vi "战舰弹窗.vi"() -> ()   [LabVIEW 2018]
panel:
  in  "关卡":dbl
  out "失败界面":picture
  out "胜利界面":picture
  out "敌机是否入侵":bool
  out "得分":dbl
  out "战舰爆炸":picture
  out "血量":dbl
  out "战舰血量":T1 scale=0.0..100.0
  out "敌机爆炸":picture
  in  "敌机数量":dbl
  in  "敌机速度":dbl
  out "敌机":picture
  out "按键":dbl
  out "战舰":T2
  out "激光武器1":T3
  out "激光武器 2":T3
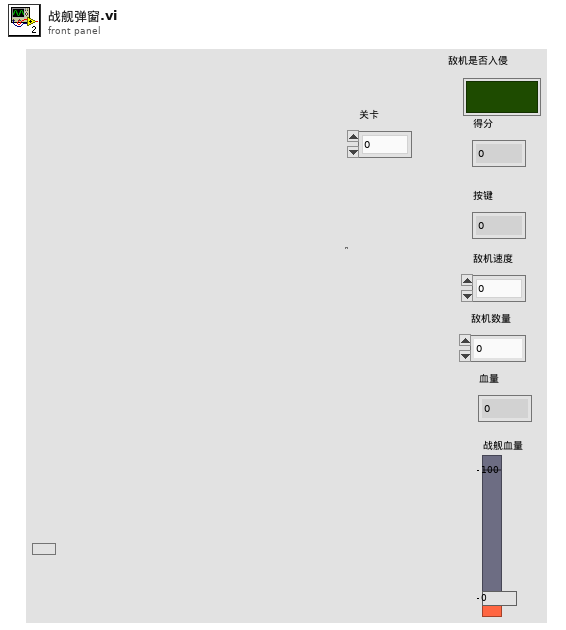
[diagram p1: front panel]
types:
  T1 = typedef "战列巡洋舰_血条.ctl" = dbl
  T2 = typedef "战列巡洋舰.ctl" = picture
  T3 = typedef "战列巡洋舰_激光武器.ctl" = picture
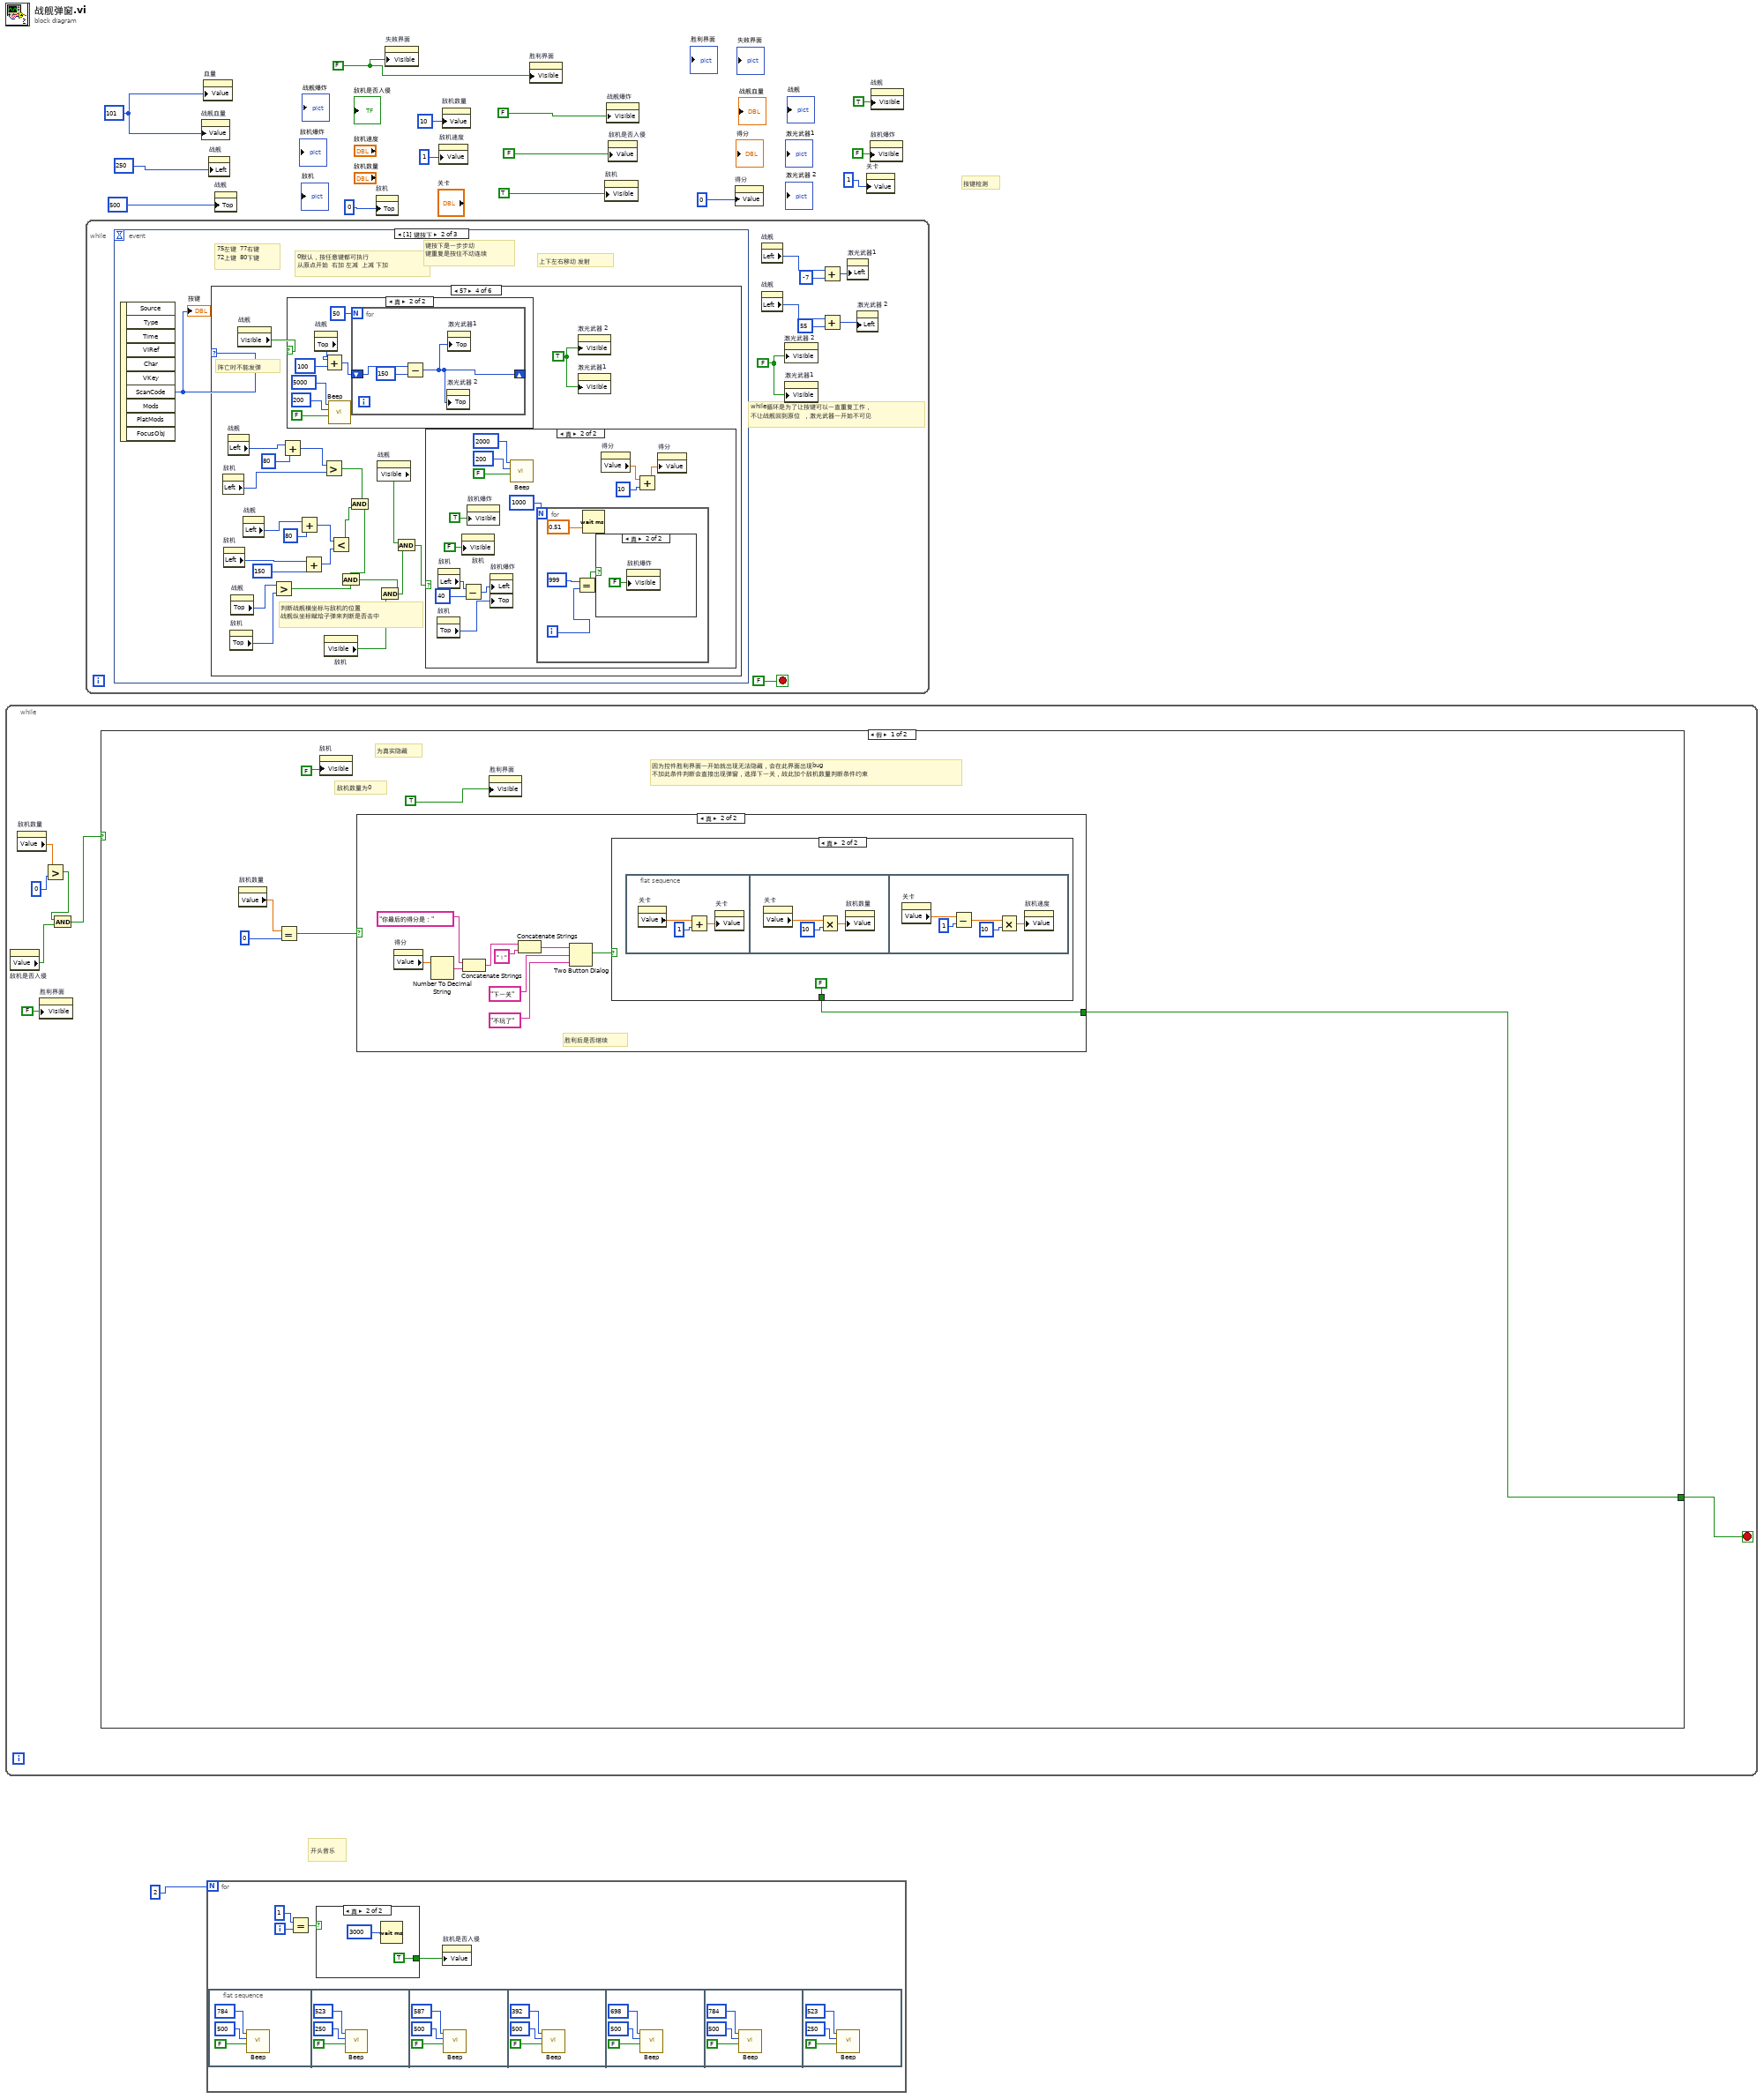
[diagram p0: block diagram]
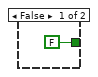
[diagram p2: hidden frame]
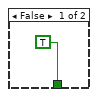
[diagram p4: hidden frame]
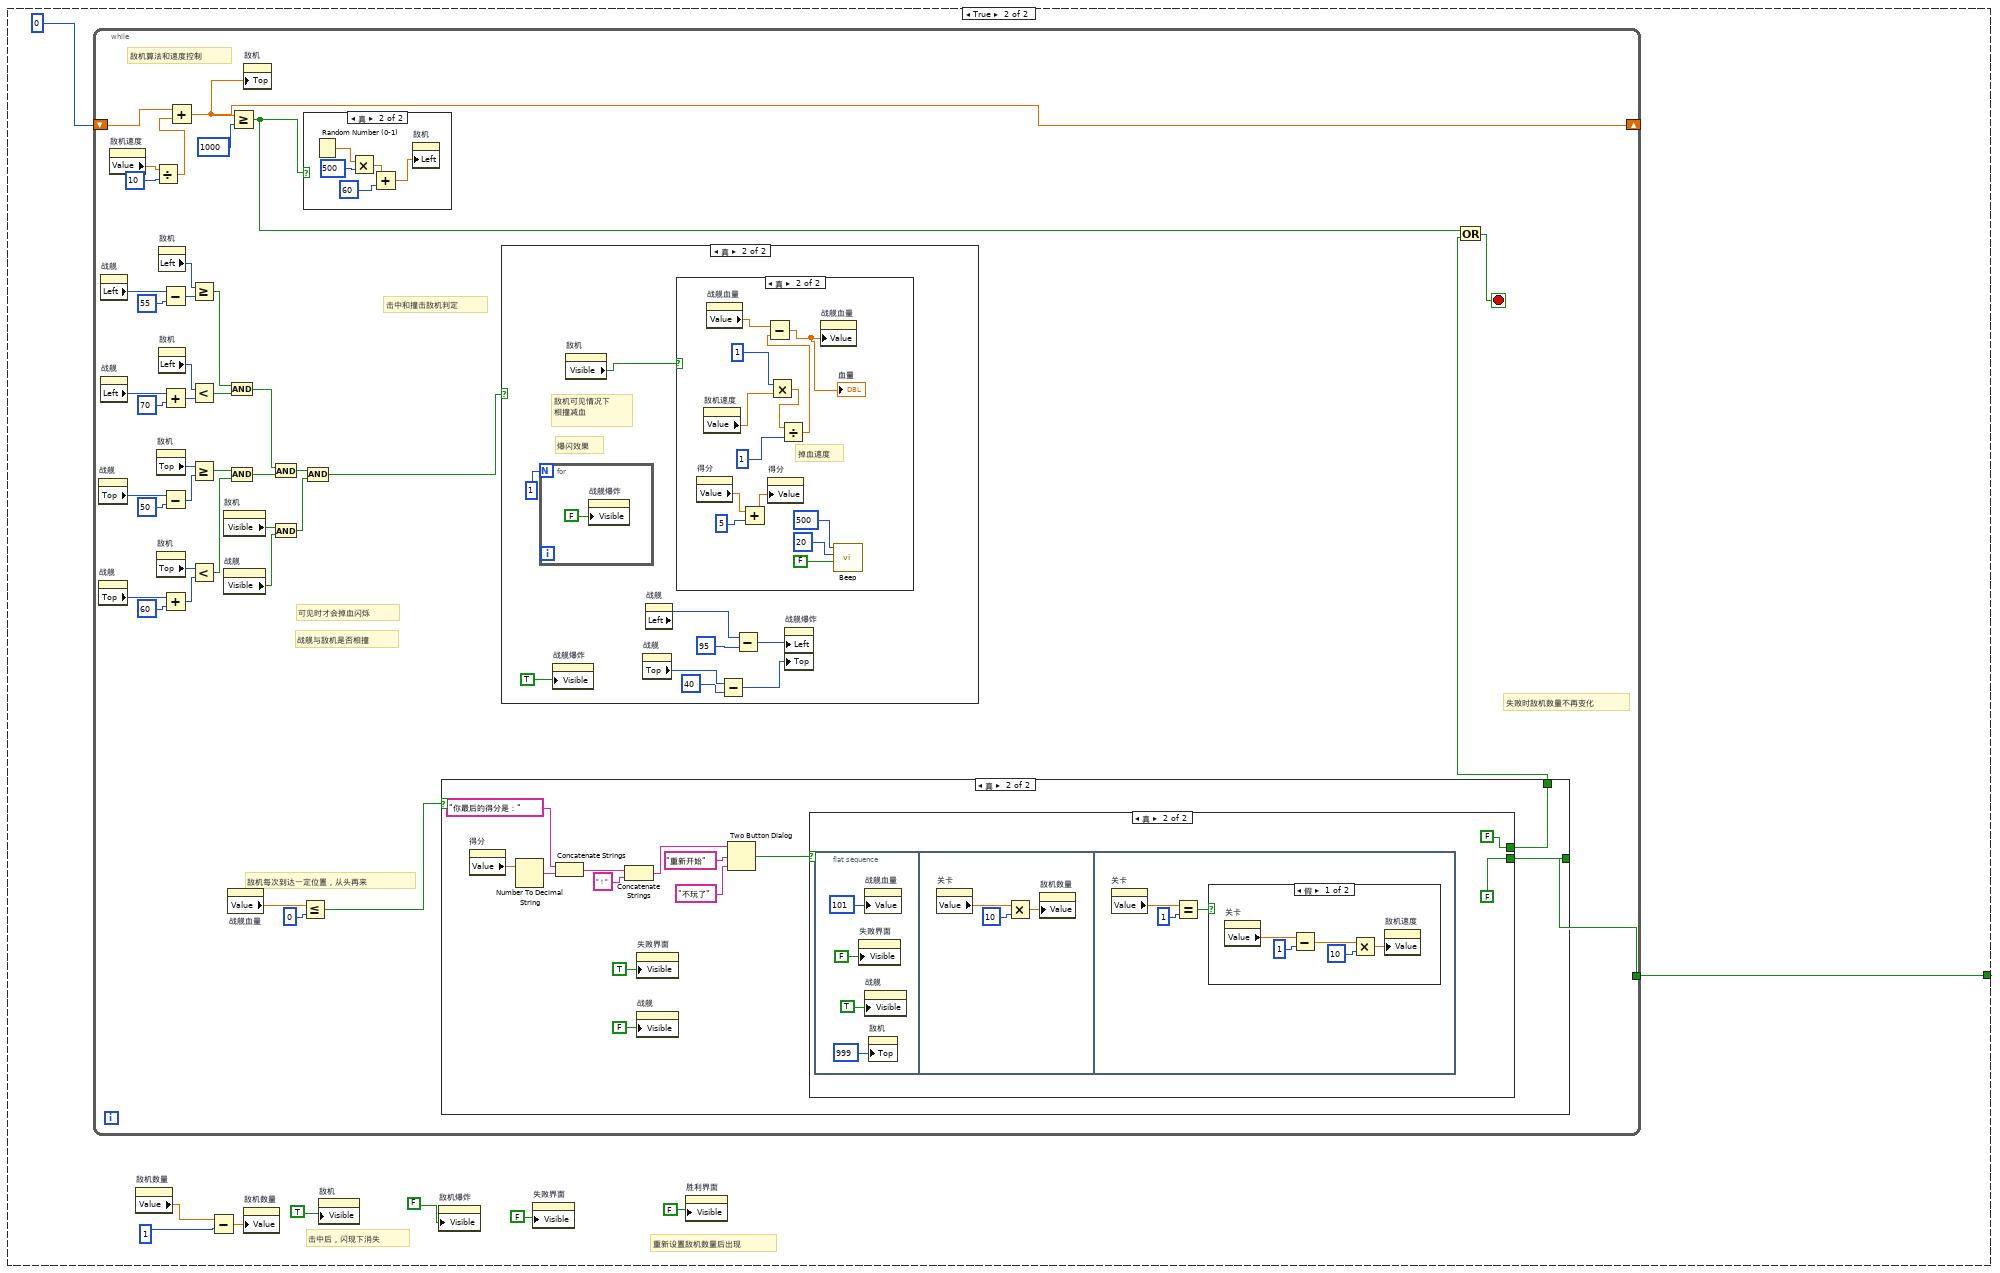
[diagram p5: hidden frame]
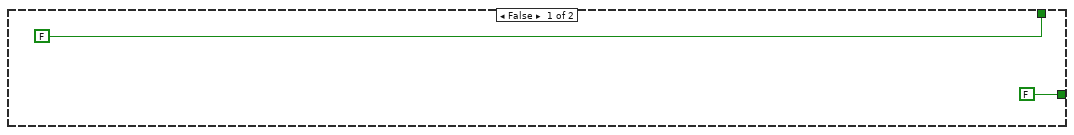
[diagram p6: hidden frame]
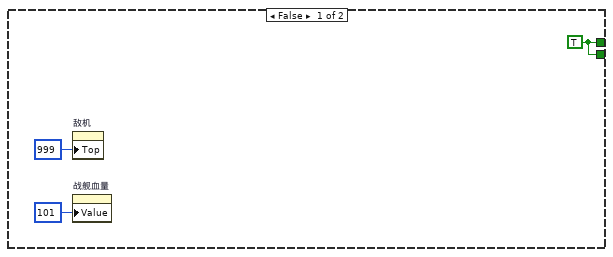
[diagram p7: hidden frame]
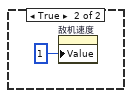
[diagram p8: hidden frame]
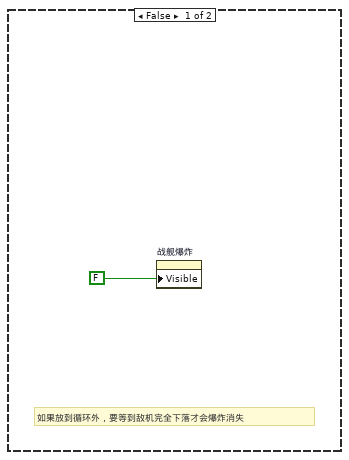
[diagram p9: hidden frame]
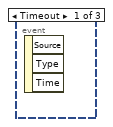
[diagram p12: hidden frame]
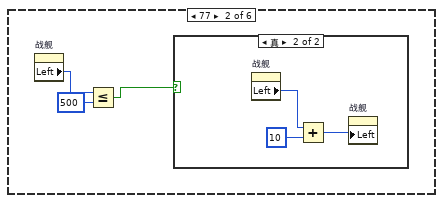
[diagram p14: hidden frame]
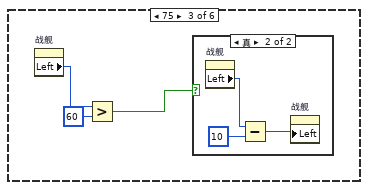
[diagram p16: hidden frame]
diagram:
  w1 = FALSE ("可见")
  w9 = 101
  # "开头音乐"
  # "按键检测"
  n1 = while {
    stop <- w17 stop-if-true
    n2 = property on="敌机是否入侵" class="Bool (严格)"() -> ("Value"=w20:bool)  [unwired: 2 in, 2 out]
    n3 = property on="敌机数量" class="DigNum (严格)"() -> ("Value"=w22:dbl)  [unwired: 2 in, 2 out]
    n4 = property on="胜利界面" class="Pict"("Visible"=FALSE ("可见")) -> ()  [unwired: 2 in, 2 out]
    n5 = Greater?(x=w22, y=0) -> (0:w19:bool)
    n6 = And(x=w19, y=w20) -> (x .and. y?=w18:bool)
    n7 = case shown="假" w18 {
      tunnel: [w26 w53] -> w17
      frame False {
        # "因为控件胜利界面一开始就出现无法隐藏，会在此界面出现bug\n不加此条件判断会直接出现弹窗，选择下一关，故此加个敌机数量判断条件约束"
        # "敌机数量为0"
        # "为真实隐藏"
        n8 = property on="敌机数量" class="DigNum (严格)"() -> ("Value"=w25:dbl)  [unwired: 2 in, 2 out]
        n9 = Equal?(x=w25, y=0) -> (x = y?=w23:bool)
        n10 = property on="敌机" class="Pict"("Visible"=FALSE ("可见")) -> ()  [unwired: 2 in, 2 out]
        n11 = case shown="真" w23 {
          tunnel: [_ w29] -> w26
          frame False {
          }
          frame True {
            # "胜利后是否继续"
            n12 = property on="得分" class="DigNum (严格)"() -> ("Value"=w37:dbl)  [unwired: 2 in, 2 out]
            n13 = Number To Decimal String(number=w37) -> (decimal integer string=w35:string)  [unwired: 1 in]
            n14 = Concatenate Strings("你最后的得分是：", w35) -> (w34:string)
            n15 = Concatenate Strings(w34, "！") -> (w32:string)
            n16 = Two Button Dialog(message=w32, 1:"不玩了" ("F按钮名称（“取消”）"), 2:"下一关" ("T按钮名称（“确定”）")) -> (T button?=w38:bool)
            n17 = case shown="真" w38 {
              tunnel: [TRUE FALSE] -> w29
              frame False {
              }
              frame True {
                n18 = flat-sequence {
                  frame #0 {
                    n19 = property on="关卡" class="DigNum (严格)"() -> ("Value"=w43:dbl)  [unwired: 2 in, 2 out]
                    n20 = Add(x=w43, y=1) -> (x+y=w41:dbl)
                    n21 = property on="关卡" class="DigNum (严格)"("Value"=w41) -> ()  [unwired: 2 in, 2 out]
                  }
                  frame #1 {
                    n22 = property on="关卡" class="DigNum (严格)"() -> ("Value"=w45:dbl)  [unwired: 2 in, 2 out]
                    n23 = Multiply(x=w45, y=10) -> (x*y=w46:dbl)
                    n24 = property on="敌机数量" class="DigNum (严格)"("Value"=w46) -> ()  [unwired: 2 in, 2 out]
                  }
                  frame #2 {
                    n25 = property on="关卡" class="DigNum (严格)"() -> ("Value"=w50:dbl)  [unwired: 2 in, 2 out]
                    n26 = Subtract(x=w50, y=1) -> (x-y=w48:dbl)
                    n27 = Multiply(x=w48, y=10) -> (x*y=w47:dbl)
                    n28 = property on="敌机速度" class="DigNum (严格)"("Value"=w47) -> ()  [unwired: 2 in, 2 out]
                  }
                }
              }
            }
          }
        }
        n29 = property on="胜利界面" class="Pict"("Visible"=TRUE ("可见")) -> ()  [unwired: 2 in, 2 out]
      }
      frame True {
        # "重新设置敌机数量后出现"
        # "击中后，闪现下消失"
        # "敌机每次到达一定位置，从头再来"
        n30 = while {
          shift-right: [w98] -> _
          shift-left: 0 -> [w100]
          tunnel: [w64] -> w53
          stop <- w62 stop-if-true
          # "失败时敌机数量不再变化"
          # "击中和撞击敌机判定"
          # "可见时才会掉血闪烁"
          # "战舰与敌机是否相撞"
          # "敌机算法和速度控制"
          n31 = property on="战舰" class="Pict (严格)"() -> ("Top"=w83:i32)  [unwired: 2 in, 2 out]
          n32 = property on="战舰" class="Pict (严格)"() -> ("Top"=w77:i32)  [unwired: 2 in, 2 out]
          n33 = property on="战舰" class="Pict (严格)"() -> ("Left"=w93:i32)  [unwired: 2 in, 2 out]
          n34 = property on="战舰" class="Pict (严格)"() -> ("Left"=w87:i32)  [unwired: 2 in, 2 out]
          n35 = property on="敌机速度" class="DigNum (严格)"() -> ("Value"=w97:dbl)  [unwired: 2 in, 2 out]
          n36 = Divide(x=w97, y=10) -> (x/y=w96:dbl)
          n37 = property on="敌机" class="Pict"() -> ("Top"=w84:i32)  [unwired: 2 in, 2 out]
          n38 = property on="敌机" class="Pict"() -> ("Top"=w76:i32)  [unwired: 2 in, 2 out]
          n39 = property on="敌机" class="Pict"() -> ("Left"=w94:i32)  [unwired: 2 in, 2 out]
          n40 = property on="敌机" class="Pict"() -> ("Left"=w89:i32)  [unwired: 2 in, 2 out]
          n41 = Subtract(x=w93, y=55) -> (x-y=w92:i32)
          n42 = Add(x=w87, y=70) -> (x+y=w86:i32)
          n43 = Subtract(x=w83, y=50) -> (x-y=w81:i32)
          n44 = Add(x=w77, y=60) -> (x+y=w79:i32)
          n45 = Add(x=w100, y=w96) -> (x+y=w98:dbl)
          n46 = Greater Or Equal?(x=w94, y=w92) -> (x >= y?=w90:bool)
          n47 = Less?(x=w89, y=w86) -> (x < y?=w85:bool)
          n48 = Greater Or Equal?(x=w84, y=w81) -> (x >= y?=w75:bool)
          n49 = Less?(x=w76, y=w79) -> (x < y?=w74:bool)
          n50 = property on="敌机" class="Pict"() -> ("Visible"=w67:bool)  [unwired: 2 in, 2 out]
          n51 = property on="战舰" class="Pict (严格)"() -> ("Visible"=w66:bool)  [unwired: 2 in, 2 out]
          n52 = And(x=w90, y=w85) -> (x .and. y?=w80:bool)
          n53 = And(x=w75, y=w74) -> (x .and. y?=w73:bool)
          n54 = property on="战舰血量" class="Slide (严格)"() -> ("Value"=w69:T1)  [unwired: 2 in, 2 out]
          n55 = Greater Or Equal?(x=w98, y=1000) -> (x >= y?=w63:bool)
          n56 = property on="敌机" class="Pict"("Top"=w98) -> ()  [unwired: 2 in, 2 out]
          n57 = And(x=w80, y=w73) -> (x .and. y?=w72:bool)
          n58 = And(x=w67, y=w66) -> (x .and. y?=w65:bool)
          n59 = Less Or Equal?(x=w69, y=0) -> (x <= y?=w70:bool)
          n60 = case shown="真" w63 {
            frame False {
            }
            frame True {
              n61 = Random Number (0-1)() -> (number: 0 to 1=w165:dbl)
              n62 = Multiply(x=w165, y=500) -> (x*y=w163:dbl)
              n63 = Add(x=w163, y=60) -> (x+y=w162:dbl)
              n64 = property on="敌机" class="Pict"("Left"=w162) -> ()  [unwired: 2 in, 2 out]
            }
          }
          n65 = And(x=w72, y=w65) -> (x .and. y?=w71:bool)
          n66 = case shown="真" w70 {
            tunnel: [FALSE w104] -> w64
            tunnel: [FALSE w103] -> w61
            frame False {
            }
            frame True {
              n67 = property on="得分" class="DigNum (严格)"() -> ("Value"=w115:dbl)  [unwired: 2 in, 2 out]
              n68 = Number To Decimal String(number=w115) -> (decimal integer string=w114:string)  [unwired: 1 in]
              n69 = Concatenate Strings("你最后的得分是：", w114) -> (w113:string)
              n70 = Concatenate Strings(w113, "！") -> (w112:string)
              n71 = property on="失败界面" class="Pict"("Visible"=TRUE ("可见")) -> ()  [unwired: 2 in, 2 out]
              n72 = property on="战舰" class="Pict (严格)"("Visible"=FALSE ("可见")) -> ()  [unwired: 2 in, 2 out]
              n73 = Two Button Dialog(message=w112, 1:"不玩了" ("F按钮名称（“取消”）"), 2:"重新开始" ("T按钮名称（“确定”）")) -> (T button?=w107:bool)
              n74 = case shown="真" w107 {
                tunnel: [w116 FALSE] -> w104
                tunnel: [w116 FALSE] -> w103
                frame False {
                  w116 = TRUE
                  n75 = property on="敌机" class="Pict"("Top"=999 ("位置:置顶")) -> ()  [unwired: 2 in, 2 out]
                  n76 = property on="战舰血量" class="Slide (严格)"("Value"=101) -> ()  [unwired: 2 in, 2 out]
                }
                frame True {
                  n77 = flat-sequence {
                    frame #0 {
                      n78 = property on="失败界面" class="Pict"("Visible"=FALSE ("可见")) -> ()  [unwired: 2 in, 2 out]
                      n79 = property on="战舰血量" class="Slide (严格)"("Value"=101) -> ()  [unwired: 2 in, 2 out]
                      n80 = property on="战舰" class="Pict (严格)"("Visible"=TRUE ("可见")) -> ()  [unwired: 2 in, 2 out]
                      n81 = property on="敌机" class="Pict"("Top"=999 ("位置:置顶")) -> ()  [unwired: 2 in, 2 out]
                    }
                    frame #1 {
                      n82 = property on="关卡" class="DigNum (严格)"() -> ("Value"=w125:dbl)  [unwired: 2 in, 2 out]
                      n83 = Multiply(x=w125, y=10) -> (x*y=w127:dbl)
                      n84 = property on="敌机数量" class="DigNum (严格)"("Value"=w127) -> ()  [unwired: 2 in, 2 out]
                    }
                    frame #2 {
                      n85 = property on="关卡" class="DigNum (严格)"() -> ("Value"=w130:dbl)  [unwired: 2 in, 2 out]
                      n86 = Equal?(x=w130, y=1) -> (x = y?=w128:bool)
                      n87 = case shown="假" w128 {
                        frame False {
                          n88 = property on="关卡" class="DigNum (严格)"() -> ("Value"=w134:dbl)  [unwired: 2 in, 2 out]
                          n89 = Subtract(x=w134, y=1) -> (x-y=w131:dbl)
                          n90 = Multiply(x=w131, y=10) -> (x*y=w135:dbl)
                          n91 = property on="敌机速度" class="DigNum (严格)"("Value"=w135) -> ()  [unwired: 2 in, 2 out]
                        }
                        frame True {
                          n92 = property on="敌机速度" class="DigNum (严格)"("Value"=1) -> ()  [unwired: 2 in, 2 out]
                        }
                      }
                    }
                  }
                }
              }
            }
          }
          n93 = case shown="真" w71 {
            frame False {
              # "如果放到循环外，要等到敌机完全下落才会爆炸消失"
              n94 = property on="战舰爆炸" class="Pict"("Visible"=FALSE ("可见")) -> ()  [unwired: 2 in, 2 out]
            }
            frame True {
              # "爆闪效果"
              # "敌机可见情况下\n相撞减血"
              n95 = for {
                N: 1 -> [_]
                n96 = property on="战舰爆炸" class="Pict"("Visible"=FALSE ("可见")) -> ()  [unwired: 2 in, 2 out]
              }
              n97 = property on="战舰爆炸" class="Pict"("Visible"=TRUE ("可见")) -> ()  [unwired: 2 in, 2 out]
              n98 = property on="敌机" class="Pict"() -> ("Visible"=w146:bool)  [unwired: 2 in, 2 out]
              n99 = property on="战舰" class="Pict (严格)"() -> ("Top"=w141:i32)  [unwired: 2 in, 2 out]
              n100 = property on="战舰" class="Pict (严格)"() -> ("Left"=w144:i32)  [unwired: 2 in, 2 out]
              n101 = case shown="真" w146 {
                frame False {
                }
                frame True {
                  # "掉血速度"
                  n102 = property on="得分" class="DigNum (严格)"() -> ("Value"=w153:dbl)  [unwired: 2 in, 2 out]
                  n103 = property on="敌机速度" class="DigNum (严格)"() -> ("Value"=w159:dbl)  [unwired: 2 in, 2 out]
                  n104 = property on="战舰血量" class="Slide (严格)"() -> ("Value"=w160:T1)  [unwired: 2 in, 2 out]
                  n105 = Add(x=w153, y=5) -> (x+y=w152:dbl)
                  n106 = Multiply(x=1, y=w159) -> (x*y=w158:dbl)
                  n107 = property on="得分" class="DigNum (严格)"("Value"=w152) -> ()  [unwired: 2 in, 2 out]
                  n108 = Divide(x=w158, y=1) -> (x/y=w155:dbl)
                  n109 = Subtract(x=w160, y=w155) -> (x-y=w154:T1)
                  "血量" <- w154
                  n110 = property on="战舰血量" class="Slide (严格)"("Value"=w154) -> ()  [unwired: 2 in, 2 out]
                  n111 = call <vilib>:"Beep.vi"("use system alert? (T)"=FALSE, "duration (msec)"=u32 20, "frequency (Hz)"=u32 500) -> ()  [unwired: 9 in]
                }
              }
              n112 = Subtract(x=w141, y=40) -> (x-y=w139:i32)
              n113 = Subtract(x=w144, y=95) -> (x-y=w142:i32)
              n114 = property on="战舰爆炸" class="Pict"("Left"=w142, "Top"=w139) -> ()  [unwired: 2 in, 2 out]
            }
          }
          n115 = Or(x=w63, y=w61) -> (x .or. y?=w62:bool)
        }
        n116 = property on="敌机数量" class="DigNum (严格)"() -> ("Value"=w58:dbl)  [unwired: 2 in, 2 out]
        n117 = Subtract(x=w58, y=1) -> (x-y=w59:dbl)
        n118 = property on="敌机数量" class="DigNum (严格)"("Value"=w59) -> ()  [unwired: 2 in, 2 out]
        n119 = property on="敌机" class="Pict"("Visible"=TRUE ("可见")) -> ()  [unwired: 2 in, 2 out]
        n120 = property on="敌机爆炸" class="Pict"("Visible"=FALSE ("可见")) -> ()  [unwired: 2 in, 2 out]
        n121 = property on="失败界面" class="Pict"("Visible"=FALSE ("可见")) -> ()  [unwired: 2 in, 2 out]
        n122 = property on="胜利界面" class="Pict"("Visible"=FALSE ("可见")) -> ()  [unwired: 2 in, 2 out]
      }
    }
  }
  n123 = while {
    stop <- FALSE stop-if-true
    w166 = FALSE
    # "while循环是为了让按键可以一直重复工作，\n不让战舰回到原位  ，激光武器一开始不可见"
    n124 = event shown="[1] 键按下" {
      selector: _ -> [_ _ _]
      dyn-events: _ -> [_ _ _]
      timeout: _ -> [_ _ _]
      event Timeout {
        n125 = event-data() -> ()  [unwired: 1 in, 3 out]
      }
      event Key Down {
        # "上下左右移动 发射"
        # "键按下是一步步动\n键重复是按住不动连续"
        # "75左键  77右键\n72上键  80下键"
        # "0默认，按任意键都可执行\n从原点开始  右加 左减  上减 下加"
        n126 = event-data() -> ("ScanCode"=w174:i16)  [unwired: 1 in, 9 out]
        "按键" <- w174
        n127 = case shown="57" w174 {
          frame 0, Default {
          }
          frame 77 {
            n128 = property on="战舰" class="Pict (严格)"() -> ("Left"=w177:i32)  [unwired: 2 in, 2 out]
            n129 = Less Or Equal?(x=w177, y=500) -> (x <= y?=w175:bool)
            n130 = case shown="真" w175 {
              frame False {
              }
              frame True {
                n131 = property on="战舰" class="Pict (严格)"() -> ("Left"=w179:i32)  [unwired: 2 in, 2 out]
                n132 = Add(x=w179, y=10) -> (x+y=w180:i32)
                n133 = property on="战舰" class="Pict (严格)"("Left"=w180) -> ()  [unwired: 2 in, 2 out]
              }
            }
          }
          frame 75 {
            n134 = property on="战舰" class="Pict (严格)"() -> ("Left"=w183:i32)  [unwired: 2 in, 2 out]
            n135 = Greater?(x=w183, y=60) -> (0:w181:bool)
            n136 = case shown="真" w181 {
              frame False {
              }
              frame True {
                n137 = property on="战舰" class="Pict (严格)"() -> ("Left"=w185:i32)  [unwired: 2 in, 2 out]
                n138 = Subtract(x=w185, y=10) -> (x-y=w186:i32)
                n139 = property on="战舰" class="Pict (严格)"("Left"=w186) -> ()  [unwired: 2 in, 2 out]
              }
            }
          }
          frame 57 {
            w209 = TRUE
            # "阵亡时不能发弹"
            # "判断战舰横坐标与敌机的位置\n战舰纵坐标赋给子弹来判断是否击中"
            n140 = property on="敌机" class="Pict"() -> ("Left"=w206:i32)  [unwired: 2 in, 2 out]
            n141 = property on="敌机" class="Pict"() -> ("Left"=w199:i32)  [unwired: 2 in, 2 out]
            n142 = property on="战舰" class="Pict (严格)"() -> ("Left"=w208:i32)  [unwired: 2 in, 2 out]
            n143 = property on="敌机" class="Pict"() -> ("Top"=w193:i32)  [unwired: 2 in, 2 out]
            n144 = property on="战舰" class="Pict (严格)"() -> ("Top"=w194:i32)  [unwired: 2 in, 2 out]
            n145 = property on="战舰" class="Pict (严格)"() -> ("Visible"=w187:bool)  [unwired: 2 in, 2 out]
            n146 = property on="战舰" class="Pict (严格)"() -> ("Left"=w201:i32)  [unwired: 2 in, 2 out]
            n147 = Greater?(x=w194, y=w193) -> (0:w195:bool)
            n148 = Add(x=w208, y=80) -> (x+y=w205:i32)
            n149 = case shown="真" w187 {
              frame False {
              }
              frame True {
                n150 = property on="战舰" class="Pict (严格)"() -> ("Top"=w215:i32)  [unwired: 2 in, 2 out]
                n151 = Add(x=w215, y=100) -> (x+y=w213:i32)
                n152 = call <vilib>:"Beep.vi"("use system alert? (T)"=FALSE, "duration (msec)"=u32 200, "frequency (Hz)"=u32 5000) -> ()  [unwired: 9 in]
                n153 = for {
                  N: 50 -> [_]
                  shift-right: [w217] -> _
                  shift-left: w213 -> [w219]
                  n154 = Subtract(x=w219, y=150) -> (x-y=w217:i32)
                  n155 = property on="激光武器 2" class="Pict (严格)"("Top"=w217) -> ()  [unwired: 2 in, 2 out]
                  n156 = property on="激光武器1" class="Pict (严格)"("Top"=w217) -> ()  [unwired: 2 in, 2 out]
                }
              }
            }
            n157 = Add(x=w201, y=80) -> (x+y=w203:i32)
            n158 = Add(x=w199, y=150) -> (x+y=w198:i32)
            n159 = Greater?(x=w205, y=w206) -> (0:w204:bool)
            n160 = property on="敌机" class="Pict"() -> ("Visible"=w191:bool)  [unwired: 2 in, 2 out]
            n161 = Less?(x=w203, y=w198) -> (x < y?=w200:bool)
            n162 = And(x=w204, y=w200) -> (x .and. y?=w196:bool)
            n163 = And(x=w196, y=w195) -> (x .and. y?=w192:bool)
            n164 = property on="战舰" class="Pict (严格)"() -> ("Visible"=w190:bool)  [unwired: 2 in, 2 out]
            n165 = And(x=w192, y=w191) -> (x .and. y?=w189:bool)
            n166 = And(x=w190, y=w189) -> (x .and. y?=w188:bool)
            n167 = case shown="真" w188 {
              frame False {
              }
              frame True {
                n168 = property on="敌机" class="Pict"() -> ("Top"=w230:i32)  [unwired: 2 in, 2 out]
                n169 = property on="敌机" class="Pict"() -> ("Left"=w228:i32)  [unwired: 2 in, 2 out]
                n170 = property on="敌机" class="Pict"("Visible"=FALSE ("可见")) -> ()  [unwired: 2 in, 2 out]
                n171 = Subtract(x=w228, y=40) -> (x-y=w227:i32)
                n172 = property on="敌机爆炸" class="Pict"("Visible"=TRUE ("可见")) -> ()  [unwired: 2 in, 2 out]
                n173 = property on="敌机爆炸" class="Pict"("Left"=w227, "Top"=w230) -> ()  [unwired: 2 in, 2 out]
                n174 = call <vilib>:"Beep.vi"("use system alert? (T)"=FALSE, "duration (msec)"=u32 200, "frequency (Hz)"=u32 2000) -> ()  [unwired: 9 in]
                n175 = for {
                  N: 1000 -> [_]
                  i -> [w235]
                  n176 = Equal?(x=999, y=w235) -> (x = y?=w236:bool)
                  n177 = Wait (ms)(milliseconds to wait=0.51) -> ()  [unwired: 1 out]
                  n178 = case shown="真" w236 {
                    frame False {
                    }
                    frame True {
                      n179 = property on="敌机爆炸" class="Pict"("Visible"=FALSE ("可见")) -> ()  [unwired: 2 in, 2 out]
                    }
                  }
                }
                n180 = property on="得分" class="DigNum (严格)"() -> ("Value"=w225:dbl)  [unwired: 2 in, 2 out]
                n181 = Add(x=w225, y=10) -> (x+y=w223:dbl)
                n182 = property on="得分" class="DigNum (严格)"("Value"=w223) -> ()  [unwired: 2 in, 2 out]
              }
            }
            n183 = property on="激光武器 2" class="Pict (严格)"("Visible"=w209) -> ()  [unwired: 2 in, 2 out]
            n184 = property on="激光武器1" class="Pict (严格)"("Visible"=w209) -> ()  [unwired: 2 in, 2 out]
          }
          frame 80 {
            n185 = property on="战舰" class="Pict (严格)"() -> ("Top"=w240:i32)  [unwired: 2 in, 2 out]
            n186 = Less?(x=w240, y=525) -> (x < y?=w238:bool)
            n187 = case shown="真" w238 {
              frame False {
              }
              frame True {
                n188 = property on="战舰" class="Pict (严格)"() -> ("Top"=w242:i32)  [unwired: 2 in, 2 out]
                n189 = Add(x=w242, y=10) -> (x+y=w241:i32)
                n190 = property on="战舰" class="Pict (严格)"("Top"=w241) -> ()  [unwired: 2 in, 2 out]
              }
            }
          }
          frame 72 {
            n191 = property on="战舰" class="Pict (严格)"() -> ("Top"=w246:i32)  [unwired: 2 in, 2 out]
            n192 = Greater Or Equal?(x=w246, y=25) -> (x >= y?=w245:bool)
            n193 = case shown="真" w245 {
              frame False {
              }
              frame True {
                n194 = property on="战舰" class="Pict (严格)"() -> ("Top"=w249:i32)  [unwired: 2 in, 2 out]
                n195 = Subtract(x=w249, y=10) -> (x-y=w248:i32)
                n196 = property on="战舰" class="Pict (严格)"("Top"=w248) -> ()  [unwired: 2 in, 2 out]
              }
            }
          }
        }
      }
      event Key Repeat {
        # "75左键  77右键\n72上键  80下键\n空格 57"
        # "0默认，按任意键都可执行\n从原点开始  右加 左减  上减 下加"
        n197 = event-data() -> ("ScanCode"=w250:i16)  [unwired: 1 in, 9 out]
        n198 = case shown="72" w250 {
          frame 0, Default {
          }
          frame 77 {
            n199 = property on="战舰" class="Pict (严格)"() -> ("Left"=w253:i32)  [unwired: 2 in, 2 out]
            n200 = Less Or Equal?(x=w253, y=500) -> (x <= y?=w252:bool)
            n201 = case shown="真" w252 {
              frame False {
              }
              frame True {
                n202 = property on="战舰" class="Pict (严格)"() -> ("Left"=w255:i32)  [unwired: 2 in, 2 out]
                n203 = Add(x=w255, y=10) -> (x+y=w256:i32)
                n204 = property on="战舰" class="Pict (严格)"("Left"=w256) -> ()  [unwired: 2 in, 2 out]
              }
            }
          }
          frame 75 {
            n205 = property on="战舰" class="Pict (严格)"() -> ("Left"=w259:i32)  [unwired: 2 in, 2 out]
            n206 = Greater Or Equal?(x=w259, y=25) -> (x >= y?=w258:bool)
            n207 = case shown="真" w258 {
              frame False {
              }
              frame True {
                n208 = property on="战舰" class="Pict (严格)"() -> ("Left"=w262:i32)  [unwired: 2 in, 2 out]
                n209 = Subtract(x=w262, y=10) -> (x-y=w261:i32)
                n210 = property on="战舰" class="Pict (严格)"("Left"=w261) -> ()  [unwired: 2 in, 2 out]
              }
            }
          }
          frame 80 {
            n211 = property on="战舰" class="Pict (严格)"() -> ("Top"=w265:i32)  [unwired: 2 in, 2 out]
            n212 = Less Or Equal?(x=w265, y=525) -> (x <= y?=w264:bool)
            n213 = case shown="真" w264 {
              frame False {
              }
              frame True {
                n214 = property on="战舰" class="Pict (严格)"() -> ("Top"=w267:i32)  [unwired: 2 in, 2 out]
                n215 = Add(x=w267, y=10) -> (x+y=w266:i32)
                n216 = property on="战舰" class="Pict (严格)"("Top"=w266) -> ()  [unwired: 2 in, 2 out]
              }
            }
          }
          frame 72 {
            n217 = property on="战舰" class="Pict (严格)"() -> ("Top"=w271:i32)  [unwired: 2 in, 2 out]
            n218 = Greater Or Equal?(x=w271, y=25) -> (x >= y?=w270:bool)
            n219 = case shown="真" w270 {
              frame False {
              }
              frame True {
                n220 = property on="战舰" class="Pict (严格)"() -> ("Top"=w274:i32)  [unwired: 2 in, 2 out]
                n221 = Subtract(x=w274, y=10) -> (x-y=w273:i32)
                n222 = property on="战舰" class="Pict (严格)"("Top"=w273) -> ()  [unwired: 2 in, 2 out]
              }
            }
          }
        }
      }
    }
    n223 = property on="战舰" class="Pict (严格)"() -> ("Left"=w172:i32)  [unwired: 2 in, 2 out]
    n224 = property on="战舰" class="Pict (严格)"() -> ("Left"=w168:i32)  [unwired: 2 in, 2 out]
    n225 = property on="激光武器 2" class="Pict (严格)"("Visible"=w166) -> ()  [unwired: 2 in, 2 out]
    n226 = property on="激光武器1" class="Pict (严格)"("Visible"=w166) -> ()  [unwired: 2 in, 2 out]
    n227 = Add(x=w172, y=-7) -> (x+y=w171:i32)
    n228 = Add(x=w168, y=55) -> (x+y=w167:i32)
    n229 = property on="激光武器1" class="Pict (严格)"("Left"=w171) -> ()  [unwired: 2 in, 2 out]
    n230 = property on="激光武器 2" class="Pict (严格)"("Left"=w167) -> ()  [unwired: 2 in, 2 out]
  }
  n231 = property on="战舰血量" class="Slide (严格)"("Value"=w9) -> ()  [unwired: 2 in, 2 out]
  n232 = property on="血量" class="DigNum (严格)"("Value"=w9) -> ()  [unwired: 2 in, 2 out]
  n233 = for {
    N: 2 -> [_]
    i -> [w276]
    n234 = flat-sequence {
      frame #0 {
        n235 = call <vilib>:"Beep.vi"("use system alert? (T)"=FALSE, "duration (msec)"=500, "frequency (Hz)"=784) -> ()  [unwired: 9 in]
      }
      frame #1 {
        n236 = call <vilib>:"Beep.vi"("use system alert? (T)"=FALSE, "duration (msec)"=250, "frequency (Hz)"=523) -> ()  [unwired: 9 in]
      }
      frame #2 {
        n237 = call <vilib>:"Beep.vi"("use system alert? (T)"=FALSE, "duration (msec)"=500, "frequency (Hz)"=587) -> ()  [unwired: 9 in]
      }
      frame #3 {
        n238 = call <vilib>:"Beep.vi"("use system alert? (T)"=FALSE, "duration (msec)"=500, "frequency (Hz)"=392) -> ()  [unwired: 9 in]
      }
      frame #4 {
        n239 = call <vilib>:"Beep.vi"("use system alert? (T)"=FALSE, "duration (msec)"=500, "frequency (Hz)"=698) -> ()  [unwired: 9 in]
      }
      frame #5 {
        n240 = call <vilib>:"Beep.vi"("use system alert? (T)"=FALSE, "duration (msec)"=500, "frequency (Hz)"=784) -> ()  [unwired: 9 in]
      }
      frame #6 {
        n241 = call <vilib>:"Beep.vi"("use system alert? (T)"=FALSE, "duration (msec)"=250, "frequency (Hz)"=523) -> ()  [unwired: 9 in]
      }
    }
    n242 = Equal?(x=1, y=w276) -> (x = y?=w278:bool)
    n243 = case shown="真" w278 {
      tunnel: [FALSE ("敌机是否入侵") TRUE ("敌机是否入侵")] -> w275
      frame False {
      }
      frame True {
        n244 = Wait (ms)(milliseconds to wait=u32 3000 ("等待时间（毫秒）")) -> ()  [unwired: 1 out]
      }
    }
    n245 = property on="敌机是否入侵" class="Bool (严格)"("Value"=w275) -> ()  [unwired: 2 in, 2 out]
  }
  n246 = property on="战舰" class="Pict (严格)"("Left"=250 ("位置:居左")) -> ()  [unwired: 2 in, 2 out]
  n247 = property on="战舰" class="Pict (严格)"("Top"=500 ("位置:置顶")) -> ()  [unwired: 2 in, 2 out]
  n248 = property on="敌机" class="Pict"("Top"=0) -> ()  [unwired: 2 in, 2 out]
  n249 = property on="失败界面" class="Pict"("Visible"=w1) -> ()  [unwired: 2 in, 2 out]
  n250 = property on="敌机速度" class="DigNum (严格)"("Value"=1) -> ()  [unwired: 2 in, 2 out]
  n251 = property on="敌机数量" class="DigNum (严格)"("Value"=10) -> ()  [unwired: 2 in, 2 out]
  n252 = property on="胜利界面" class="Pict"("Visible"=w1) -> ()  [unwired: 2 in, 2 out]
  n253 = property on="敌机" class="Pict"("Visible"=TRUE ("可见")) -> ()  [unwired: 2 in, 2 out]
  n254 = property on="战舰爆炸" class="Pict"("Visible"=FALSE ("可见")) -> ()  [unwired: 2 in, 2 out]
  n255 = property on="敌机是否入侵" class="Bool (严格)"("Value"=FALSE ("敌机是否入侵")) -> ()  [unwired: 2 in, 2 out]
  n256 = property on="得分" class="DigNum (严格)"("Value"=0) -> ()  [unwired: 2 in, 2 out]
  n257 = property on="关卡" class="DigNum (严格)"("Value"=1) -> ()  [unwired: 2 in, 2 out]
  n258 = property on="敌机爆炸" class="Pict"("Visible"=FALSE ("可见")) -> ()  [unwired: 2 in, 2 out]
  n259 = property on="战舰" class="Pict (严格)"("Visible"=TRUE ("可见")) -> ()  [unwired: 2 in, 2 out]
